vi "DeviceCodeToEccType.vi"(5 "Device Code":i32) -> (2 "EccType":enum16{"ecc", "ecc4", "ecc5"}(ring))   [LabVIEW 2022 SP3, in "EClib functions.lvlib"]
uses:
  EClib functions.lvlib
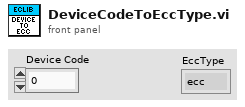
[diagram p1: front panel]
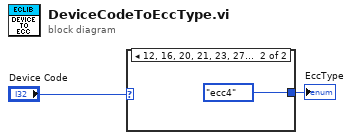
[diagram p0: block diagram]
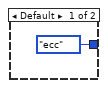
[diagram p2: hidden frame]
diagram:
  n1 = case shown="12, 16, 20, 21, 23, 27, 32" "Device Code" {
    tunnel: [enum16{"ecc", "ecc4"}."ecc" enum16{"ecc", "ecc4"}."ecc4"] -> w1
    frame Default {
    }
    frame 12, 16, 20, 21, 23, 27, 32 {
    }
  }
  "EccType" <- w1
